vi "DHE_CheckBusy.vi"(8 "error in (no error)":errorcluster, 9 "command":string, 10 "timeout (2000 ms)":u32=2000) -> (0 "error out":errorcluster, 2 "busy?":bool)   [LabVIEW 2016]
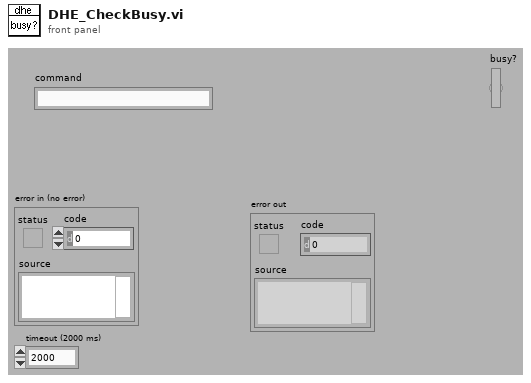
[diagram p1: front panel]
types:
  T1 = enum16{"Idle", "Exposing", "Paused", "AbortExp", "Reading", "AbortRead", "FinishedReading", "Resetting", "Reducing", "Initializing"}
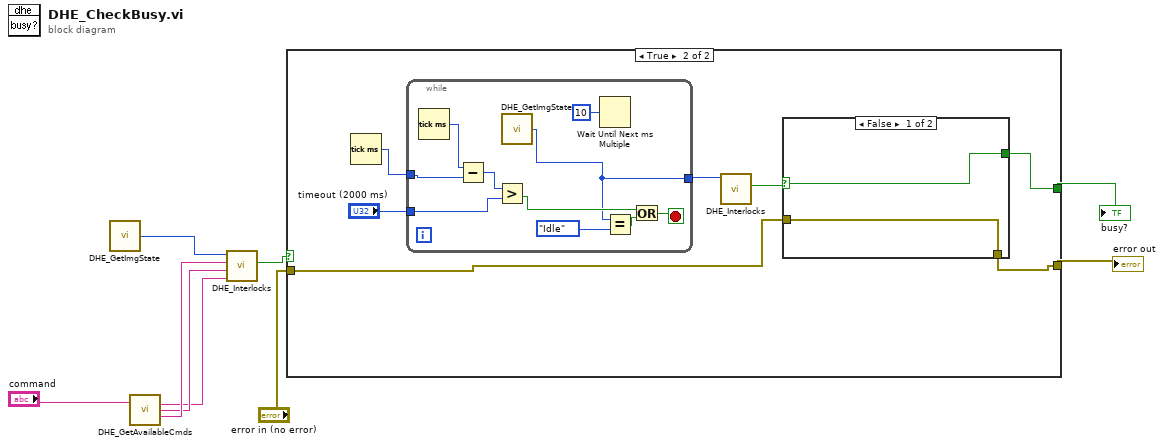
[diagram p0: block diagram]
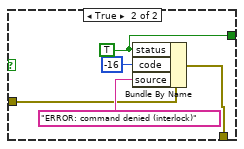
[diagram p3: hidden frame]
diagram:
  n1 = call "DHE_GetImgState.vi"() -> ("DHE_ImgState"=w1:T1)  [unwired: 9 out]
  n2 = call "DHE_GetAvailableCmds.vi"("input command"="command") -> ("remaining"=w2:string, "field"=w4:string, "parent"=w5:string)  [unwired: 12 out]
  n3 = call "DHE_Interlocks.vi"("remaining"=w2, "field"=w4, "parent"=w5, "DHE_ImgState"=w1) -> ("interlock closed"=w3:bool)  [unwired: 7 out]
  n4 = case shown="True" w3 {
    selector: w3 -> [w10 _]
    tunnel: [w11 w13] -> w9
    tunnel: [w10 w12] -> w8
    tunnel: "error in (no error)" -> [w11 w14]
    frame False {
    }
    frame True {
      n5 = Tick Count (ms)() -> (millisecond timer value=w17:u32)
      n6 = while {
        tunnel: [w27] -> w16
        tunnel: w17 -> [w33]
        tunnel: "timeout (2000 ms)" -> [w29]
        stop <- w28 stop-if-true
        n7 = Tick Count (ms)() -> (millisecond timer value=w34:u32)
        n8 = Subtract(x=w34, y=w33) -> (x-y=w31:u32)
        n9 = Greater?(x=w31, y=w29) -> (0:w30:bool)
        n10 = call "DHE_GetImgState.vi"() -> ("DHE_ImgState"=w27:T1)  [unwired: 9 out]
        n11 = Wait Until Next ms Multiple(millisecond multiple=u32 10) -> ()  [unwired: 1 out]
        n12 = Equal?(x=w27, y=T1."Idle" ("DHE_ImgState")) -> (x = y?=w32:bool)
        n13 = Or(x=w30, y=w32) -> (x .or. y?=w28:bool)
      }
      n14 = call "DHE_Interlocks.vi"("DHE_ImgState"=w16) -> ("interlock closed"=w15:bool)  [unwired: 3 in, 7 out]
      n15 = case shown="False" w15 {
        selector: w15 -> [w20 _]
        tunnel: w14 -> [w19 w23]
        tunnel: [w19 w22] -> w13
        tunnel: [w20 w21] -> w12
        frame False {
        }
        frame True {
          w21 = TRUE ("status")
          n16 = Bundle By Name(cluster=w23, "status"=w21, "code"=-16, "source"="ERROR: command denied (interlock)") -> (w22:errorcluster)
        }
      }
    }
  }
  "error out" <- w9
  "busy?" <- w8
